vi "FeedbackDecode_BuildLocalPath.vi"(0 "DataDir":string, 1 "FilePattern":string caption="pattern (all files)", 5 "DataFolder":string, 9 "HeaderName":string caption="pattern (all files)", 11 "ErrorIn":errorcluster) -> (4 "OriginalName":path, 8 "NewLocalName":path, 10 "FileExt":string, 15 "ErrorOut":errorcluster)   [LabVIEW 2020]
uses:
  <vilib>/regexp/Match Regular Expression.xnode
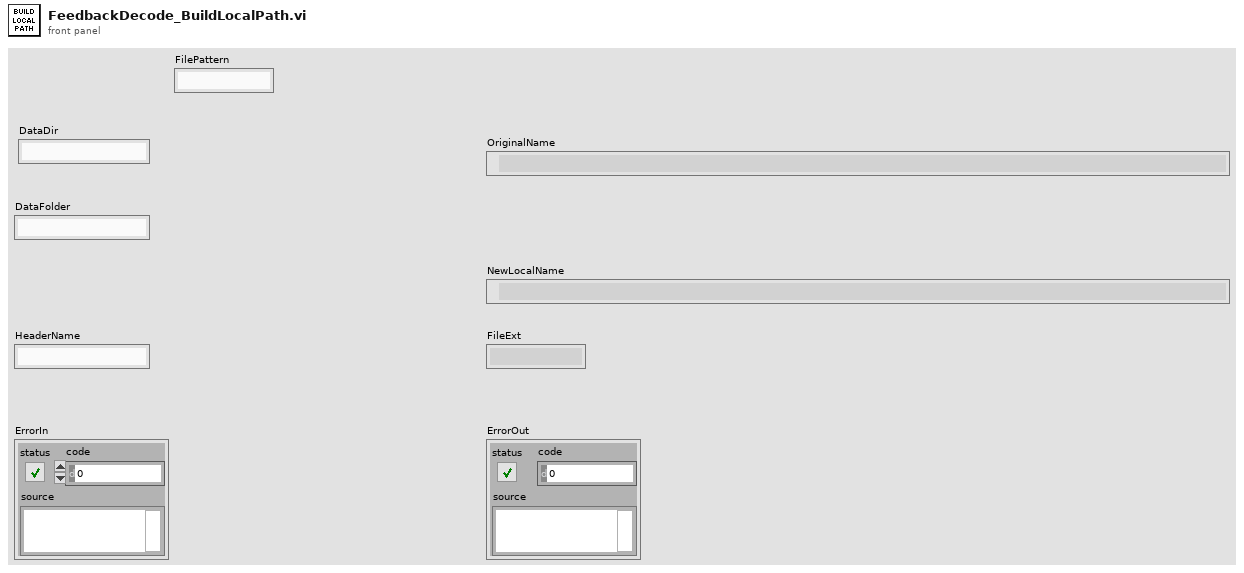
[diagram p1: front panel]
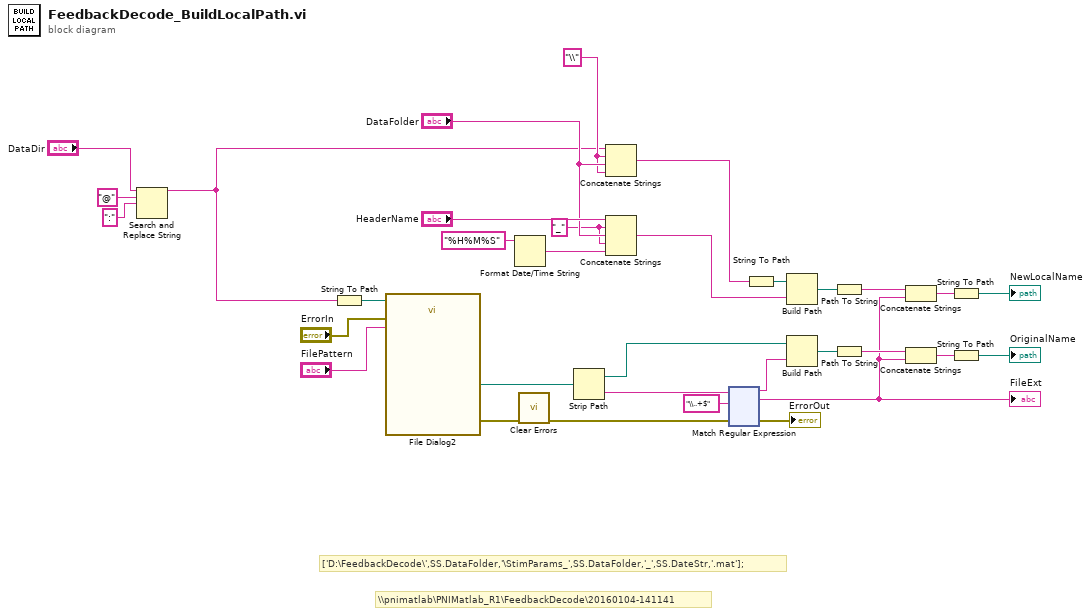
[diagram p0: block diagram]
diagram:
  w6 = "\\" ("input string")
  w29 = "_" ("string")
  # "['D:\\FeedbackDecode\\',SS.DataFolder,'\\StimParams_',SS.DataFolder,'_',SS.DateStr,'.mat'];"
  # "\\\\pnimatlab\\PNIMatlab_R1\\FeedbackDecode\\20160104-141141"
  n1 = Search and Replace String(input string="DataDir", search string="@", replace string=":" ("replace string (\"\")")) -> (result string=w1:string)  [unwired: 5 in, 3 out]
  n2 = String To Path(string=w1) -> (path=w5:path)
  n3 = call "File Dialog2"("start path"=w5, "error in"="ErrorIn", "pattern (all files)"="FilePattern") -> ("selected path"=w24:path, "error out"=w10:errorcluster)  [unwired: 9 in, 2 out]
  n4 = Format Date/Time String(time format string (%c)="%H%M%S") -> (date/time string=w28:string)  [unwired: 2 in]
  n5 = call <vilib>:"Clear Errors.vi"("error in (no error)"=w10) -> ("error out"=w9:errorcluster)  [unwired: 5 in, 1 out]
  n6 = Strip Path(path=w24) -> (stripped path=w20:path, name=w23:string)
  n7 = Concatenate Strings(w1, w6, "DataFolder", w6) -> (w26:string)
  n8 = Concatenate Strings("HeaderName", w29, "DataFolder", w29, w28) -> (w25:string)
  n9 = xnode "Match Regular Expression"("input string"=w23, "regular expression"="\\..+$", "error in"=w9) -> ("before match"=w21:string, "whole match"=w13:string, "error out"=→"ErrorOut":errorcluster)  [unwired: 3 in, 2 out]
  "FileExt" <- w13
  n10 = String To Path(string=w26) -> (path=w27:path)
  n11 = Build Path(base path=w27, name or relative path=w25) -> (appended path=w17:path)
  n12 = Build Path(base path=w20, name or relative path=w21) -> (appended path=w15:path)
  n13 = Path To String(path=w17) -> (string=w16:string)
  n14 = Path To String(path=w15) -> (string=w14:string)
  n15 = Concatenate Strings(w16, w13) -> (w19:string)
  n16 = Concatenate Strings(w14, w13) -> (w18:string)
  n17 = String To Path(string=w19) -> (path=→"NewLocalName":path)
  n18 = String To Path(string=w18) -> (path=→"OriginalName":path)
